vi "get last register.vi"(11 "Modbus Module Channel in":refnum<class "Modbus Module Channel.lvclass">) -> (3 "last element":i32)   [LabVIEW 2013, in "Modbus Module Channel.lvclass"]
uses:
  Modbus Module Channel.lvclass
  <vilib>/NI/Tag Bus/tag/tag descriptor.lvclass/tag descriptor.ctl
  Modbus Module Channel.lvclass/Modbus Module Channel.ctl
  <vilib>/NI/Tag Bus/tag/tag descriptor.lvclass
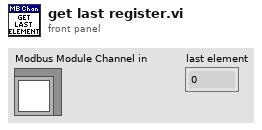
[diagram p1: front panel]
types:
  T1 = typedef "Modbus Module Channel.lvclass/data bank type.ctl" = enum16{"coils", "discrete inputs", "input registers", "holding registers"}
  T2 = typedef "tag bus.lvlib/tag descriptor.lvclass/Data Type.ctl" = enum16{"Double", "Single", "I64", "I32", "I16", "I8", "U64", "U32", "U16", "U8", "Boolean", "String", "Array of Double", "Array of Single", "Array of I64", "Array of I32", "Array of I16", "Array of I8", "Array of U64", "Array of U32", "Array of U16", "Array of U8", "Array of Boolean", "Array of String"}
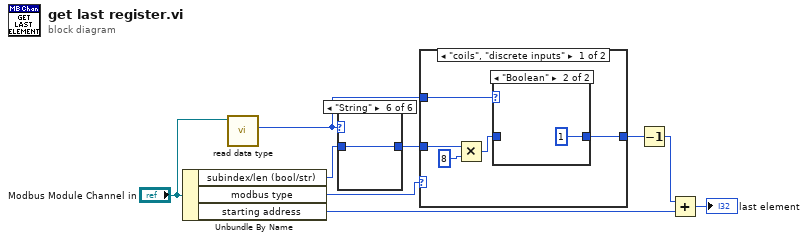
[diagram p0: block diagram]
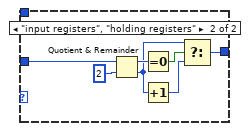
[diagram p3: hidden frame]
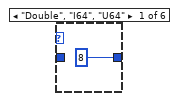
[diagram p4: hidden frame]
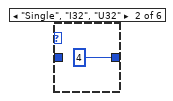
[diagram p5: hidden frame]
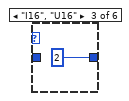
[diagram p6: hidden frame]
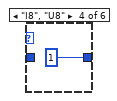
[diagram p7: hidden frame]
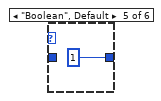
[diagram p8: hidden frame]
diagram:
  n1 = Unbundle By Name("Modbus Module Channel in") -> ("subindex/len (bool/str)"=w1:i32, "modbus type"=w5:T1, "starting address"=w9:u16)
  n2 = call <vilib>:"read data type.vi"("system tag in"="Modbus Module Channel in") -> ("data type"=w3:T2)  [unwired: 8 in, 2 out]
  n3 = case shown="\"String\"" w3 {
    tunnel: [8 ("x") 4 ("x") 2 ("x") 1 ("x") 1 ("x") w15] -> w6
    tunnel: w1 -> [_ _ _ _ _ w15]
    frame "Double", "I64", "U64" {
    }
    frame "Single", "I32", "U32" {
    }
    frame "I16", "U16" {
    }
    frame "I8", "U8" {
    }
    frame "Boolean", Default {
    }
    frame "String" {
    }
  }
  n4 = case shown="\"coils\", \"discrete inputs\"" w5 {
    tunnel: w6 -> [w20 w29]
    tunnel: [w17 w23] -> w4
    tunnel: w3 -> [w18 _]
    frame "coils", "discrete inputs" {
      n5 = Multiply(x=w20, y=8) -> (x*y=w16:i32)
      n6 = case shown="\"Boolean\"" w18 {
        tunnel: [w21 1] -> w17
        tunnel: w16 -> [w21 _]
        frame Default {
        }
        frame "Boolean" {
        }
      }
    }
    frame "input registers", "holding registers" {
      n7 = Quotient & Remainder(x=w29, y=2) -> (x-y*floor(x/y)=w27:i32, floor(x/y)=w25:i32)
      n8 = Equal To 0?(x=w27) -> (x = 0?=w26:bool)
      n9 = Increment(x=w25) -> (x+1=w24:i32)
      n10 = Select(t=w25, s=w26, f=w24) -> (s? t:f=w23:i32)
    }
  }
  n11 = Decrement(x=w4) -> (x-1=w2:i32)
  n12 = Add(x=w2, y=w9) -> (x+y=→"last element":i32)
